vi "cDAQ DDS Test Panel.vi"(8 "error in":errorcluster, 11 "cDAQ dds":T1={"device"="", "channels"=[], "mclk source"="", "mclk [Hz]"=0.0, "fs [Hz]"=0.0, "block [s]"=0.0, "buf [s]"=0.0, "task"="", "cmd queue"=refnum, "proc ref"=refnum, "smpl clock out"="/cDAQ3/PFI0", "export smpl clock"=FALSE, "DC ofs [V]"=[], "timebase source"="", "timebase mode"=enum."Local", "dither"=enum."Disabled", "dither level"=0.0, "phase [rad]"=[]} {"channels" min=0 step=1}) -> (0 "error out":errorcluster, 3 "cDAQ dds out":T1={"device"="", "channels"=[], "mclk source"="", "mclk [Hz]"=0.0, "fs [Hz]"=0.0, "block [s]"=0.0, "buf [s]"=0.0, "task"="", "cmd queue"=refnum, "proc ref"=refnum, "smpl clock out"="/cDAQ3/PFI0", "export smpl clock"=FALSE, "DC ofs [V]"=[], "timebase source"="", "timebase mode"=enum."Local", "dither"=enum."Disabled", "dither level"=0.0, "phase [rad]"=[]} {"channels" min=0 step=1})   [LabVIEW 2020]
uses:
  cDAQ DDS Session.ctl
  cDAQ DDS Setup.ctl
  cDAQ DDS Timebase Mode.ctl
  cDAQ DDS Dither.ctl
panel:
  out "DDS process is running":bool
  out "idn string":string
  in  "Phases [deg]":dbl[](array[slide]) scale=-180.0..180.0
  in  "Amplitudes [V]":dbl[](array[slide]) scale=1e-06..4.2 scale format="%#_6p"
  in  "f [Hz]":dbl=50.0
  in  "btn ok":bool caption="OK Button"
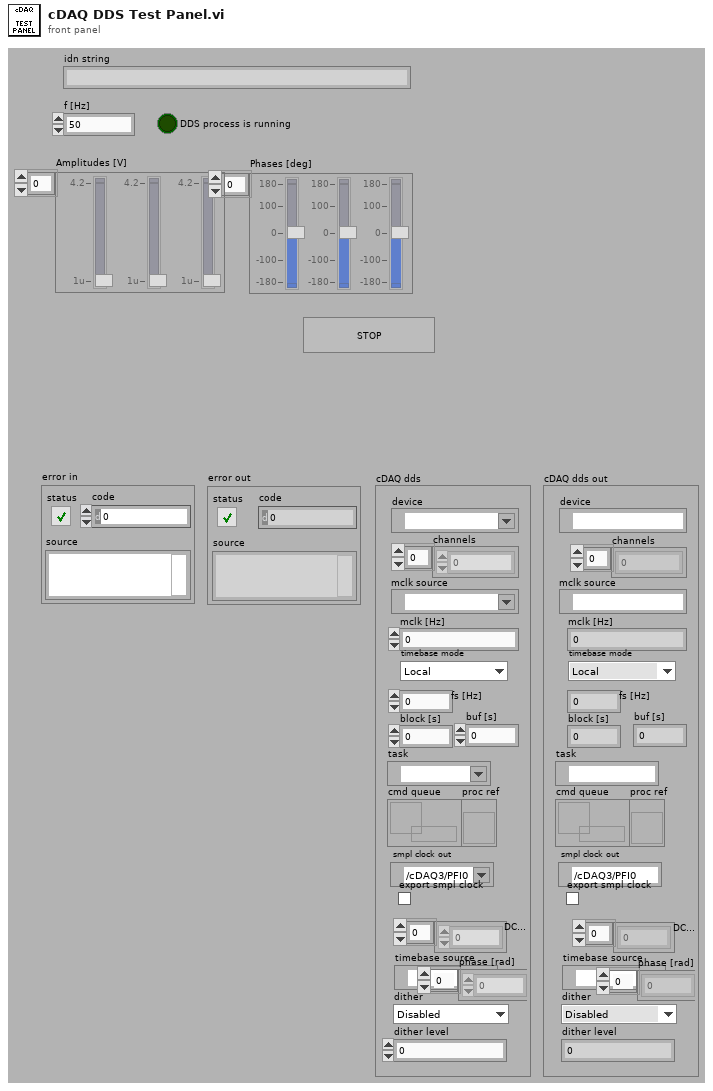
[diagram p1: front panel]
types:
  T1 = typedef "cDAQ DDS Session.ctl" = cluster{"device":tag, "channels":i32[], "mclk source":tag, "mclk [Hz]":dbl, "fs [Hz]":dbl, "block [s]":dbl, "buf [s]":dbl, "task":refnum<k21>, "cmd queue":refnum<queue>, "proc ref":refnum<vi>, "smpl clock out":tag, "export smpl clock":bool, "DC ofs [V]":dbl[], "timebase source":tag, "timebase mode":T2, "dither":T3, "dither level":dbl, "phase [rad]":dbl[]}
  T2 = typedef "cDAQ DDS Timebase Mode.ctl" = enum16{"Local", "Take from ADC (e.g. NI 9238)", "Other source"}
  T3 = typedef "cDAQ DDS Dither.ctl" = enum16{"Disabled", "Gaussian"}
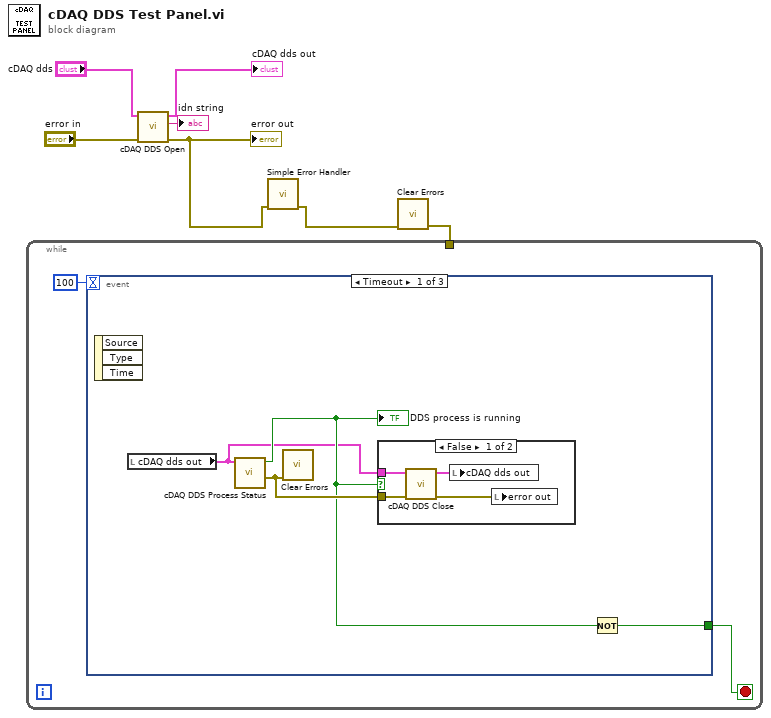
[diagram p0: block diagram]
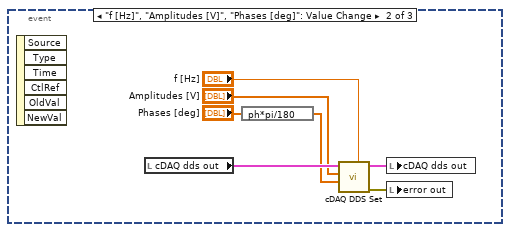
[diagram p3: hidden frame]
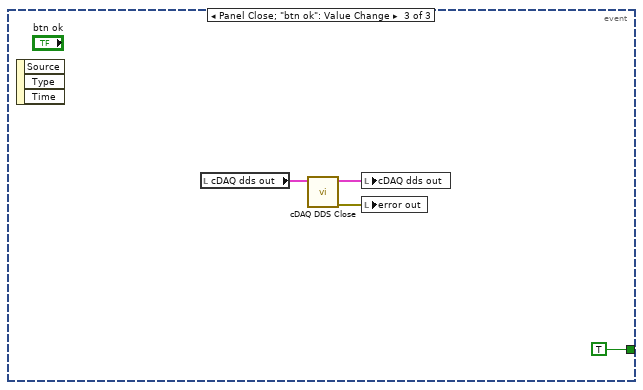
[diagram p4: hidden frame]
diagram:
  n1 = call "cDAQ DDS Open.vi"("error in"="error in", "session in"="cDAQ dds") -> ("error out"=w2:errorcluster, "idn string"=→"idn string":string, "session out"=→"cDAQ dds out":T1)  [unwired: 7 in]
  "error out" <- w2
  n2 = call <vilib>:"Simple Error Handler.vi"("error in (no error)"=w2) -> ("error out"=w1:errorcluster)  [unwired: 4 in, 4 out]
  n3 = call <vilib>:"Clear Errors.vi"("error in (no error)"=w1) -> ("error out"=w3:errorcluster)  [unwired: 5 in, 1 out]
  n4 = while {
    tunnel: w3 -> [_]
    stop <- w9 stop-if-true
    n5 = event shown="[0] Timeout" {
      selector: _ -> [_ _ _]
      dyn-events: _ -> [_ _ _]
      timeout: 100 -> [_ _ _]
      tunnel: [w10 _ TRUE] -> w9
      event Timeout {
        n6 = event-data() -> ()  [unwired: 1 in, 3 out]
        n7 = local read "cDAQ dds out"() -> (w11:T1)
        n8 = call "cDAQ DDS Process Status.vi"("cDAQ dds"=w11) -> ("sweep error out"=w13:errorcluster, "is running"=w12:bool)  [unwired: 8 in, 1 out]
        "DDS process is running" <- w12
        n9 = call <vilib>:"Clear Errors.vi"("error in (no error)"=w13) -> ()  [unwired: 5 in, 2 out]
        n10 = case shown="False" w12 {
          tunnel: w13 -> [w17 _]
          tunnel: w11 -> [w16 _]
          frame False {
            n11 = call "cDAQ DDS Close.vi"("error in"=w17, "cdaq session in"=w16) -> ("error out"=w15:errorcluster, "cdaq session out"=w14:T1)  [unwired: 8 in]
            n12 = local write "cDAQ dds out"(w14) -> ()
            n13 = local write "error out"(w15) -> ()
          }
          frame True {
          }
        }
        n14 = Not(x=w12) -> (.not. x?=w10:bool)
      }
      event "f [Hz]", "Amplitudes [V]", "Phases [deg]": Value Change {
        n15 = event-data() -> ()  [unwired: 1 in, 6 out]
        n16 = local read "cDAQ dds out"() -> (w24:T1)
        n17 = expression code="ph*pi/180"("Phases [deg]") -> (w18:dbl[])
        n18 = call "cDAQ DDS Set.vi"("common f [Hz]"="f [Hz]", "ph [rad]"=w18, "A [V]"="Amplitudes [V]", "cDAQ dds"=w24) -> ("error out"=w20:errorcluster, "cDAQ dds out"=w19:T1)  [unwired: 6 in]
        n19 = local write "cDAQ dds out"(w19) -> ()
        n20 = local write "error out"(w20) -> ()
      }
      event Panel Close; "btn ok": Value Change {
        n21 = event-data() -> ()  [unwired: 1 in, 3 out]
        n22 = local read "cDAQ dds out"() -> (w26:T1)
        n23 = call "cDAQ DDS Close.vi"("cdaq session in"=w26) -> ("error out"=w27:errorcluster, "cdaq session out"=w25:T1)  [unwired: 9 in]
        n24 = local write "cDAQ dds out"(w25) -> ()
        n25 = local write "error out"(w27) -> ()
      }
    }
  }
